vi "Font Color.vi"(8 "error in (no error)":errorcluster, 11 "Valve Item in":refnum<class "Valve Item.lvclass">) -> (0 "error out":errorcluster, 2 "Font Color":u32(colorbox), 3 "Valve Item out":refnum<class "Valve Item.lvclass">)   [LabVIEW 2020, in "BetterDragAndDropDemo.lvlib" / "Valve Item.lvclass"]
uses:
  Valve Item.lvclass
  Valve Item.lvclass/Valve Item.ctl
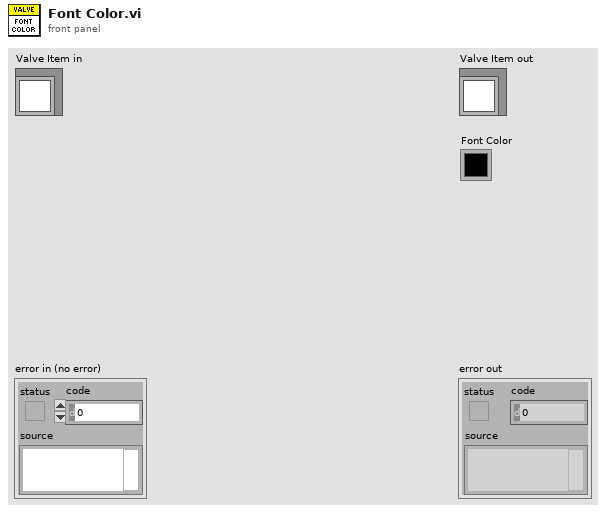
[diagram p1: front panel]
types:
  T1 = typedef "BetterDragAndDropDemo.lvlib/Valve Item.lvclass/valve color.ctl" = enum16{"black", "red"}
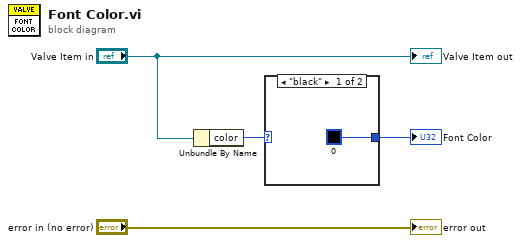
[diagram p0: block diagram]
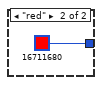
[diagram p2: hidden frame]
diagram:
  n1 = Unbundle By Name("Valve Item in") -> ("color"=w1:T1)
  n2 = case shown="\"black\"" w1 {
    tunnel: [u32 0 u32 16711680] -> w3
    frame "black" {
    }
    frame "red" {
    }
  }
  "Font Color" <- w3
  "error out" <- "error in (no error)"
  "Valve Item out" <- "Valve Item in"
